vi "DSF.Engine.Framework.Allocate Intermediate Buffer.vi"(8 "error in (no error)":errorcluster, 10 "unallocated Intermediate Buffer":refnum<class "DSF.Engine.Pointer.DBL.lvclass">, 11 "Framework in":refnum<class "VeriStand DSF.Framework.lvclass">) -> (0 "error out":errorcluster, 2 "allocated Intermediate Buffer":refnum<class "DSF.Engine.Pointer.DBL.lvclass">, 3 "Framework out":refnum<class "VeriStand DSF.Framework.lvclass">)   [LabVIEW 2017, in "Data Sharing Framework Engine.lvlib" / "VeriStand DSF.Framework.lvclass"]
uses:
  VeriStand DSF.Framework.lvclass
  DSF Core/Built/PharLap x86/Engine/c/DSF.Engine.lvlibp/Engine/Classes/Pointer/DSF.Engine.Pointer.DBL.lvclass
  DSF Core/Built/PharLap x86/Engine/c/DSF.Engine.lvlibp/Engine/Classes/Framework/DSF.Engine.Framework.lvclass
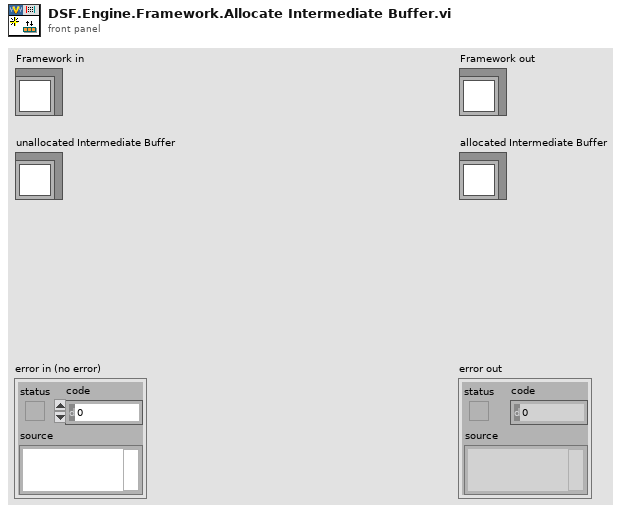
[diagram p1: front panel]
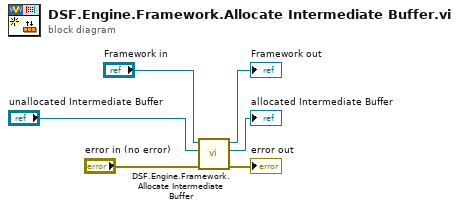
[diagram p0: block diagram]
diagram:
  n1 = call-parent "DSF.Engine.Framework.Allocate Intermediate Buffer.vi"("error in (no error)"="error in (no error)", "unallocated Intermediate Buffer"="unallocated Intermediate Buffer", "Framework in"="Framework in") -> ("error out"=→"error out":errorcluster, "allocated Intermediate Buffer"=→"allocated Intermediate Buffer":refnum<class "DSF.Engine.Pointer.DBL.lvclass">, "Framework out"=→"Framework out":refnum<class "VeriStand DSF.Framework.lvclass">)  [unwired: 6 in]
